vi "Reset.vi"(8 "error in (no error)":errorcluster, 11 "VISA resource name":refnum<visa-resource-name>) -> (0 "error out":errorcluster, 3 "VISA resource name out":refnum<visa-resource-name>)   [LabVIEW 2023, in "Thermotron 8800.lvlib"]
doc: "Resets the instrument and then sends a set of default setup commands to the instrument."
uses:
  Thermotron 8800.lvlib
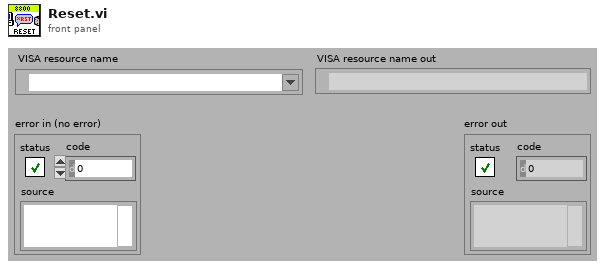
[diagram p1: front panel]
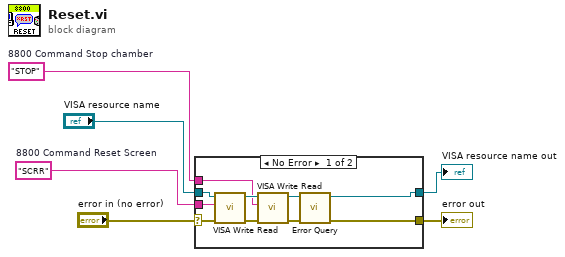
[diagram p0: block diagram]
diagram:
  w3 = "STOP"  # 8800 Command Stop chamber
  w5 = "SCRR"  # 8800 Command Reset Screen
  n1 = case shown="No Error" "error in (no error)" {
    selector: "error in (no error)" -> [w7 w18]
    tunnel: w5 -> [w12 _]
    tunnel: "VISA resource name" -> [w11 w17]
    tunnel: w3 -> [w10 _]
    tunnel: [w9 w18] -> w2
    tunnel: [w8 w17] -> w1
    frame No Error {
      n2 = call "VISA Write Read.vi"("error in (no error)"=w7, "8800 Command"=w12, "VISA Refnum in"=w11) -> ("error out"=w14:errorcluster, "VISA Refnum out"=w13:refnum<visa-resource-name>)  [unwired: 6 in, 1 out]
      n3 = call "VISA Write Read.vi"("error in (no error)"=w14, "8800 Command"=w10, "VISA Refnum in"=w13) -> ("error out"=w16:errorcluster, "VISA Refnum out"=w15:refnum<visa-resource-name>)  [unwired: 6 in, 1 out]
      n4 = call "Error Query.vi"("error in (no error)"=w16, "VISA resource name"=w15) -> ("error out"=w9:errorcluster, "VISA resource name out"=w8:refnum<visa-resource-name>)  [unwired: 6 in, 2 out]
    }
    frame Error {
      # "execute no code if incoming error"
    }
  }
  "error out" <- w2
  "VISA resource name out" <- w1
